vi "CPP-5168-SurfaceCp-Jan2013.vi"() -> (5 "Plug in titles":string[](array[string]), 7 "Plug in values":string[](array[string]))   [LabVIEW 2012]
uses:
  Globals/Meas_global.vi
panel:
  in  "inH20/V":dbl=2.4377 caption="Calibration factor inH20/V"
  in  "Last non-pressure channel":string="HW (HF3)"
  out "Zeroes?":bool
  out "Zeroes":dbl[](array[numeric])
  out "Data":dbl[][](array[numeric]) caption="ZeroedCompensatedCalibratedData" format="%#_3g"
  out "ChannelNames":string[](array[string])
  # "This version doesn't do any window dP calculations"
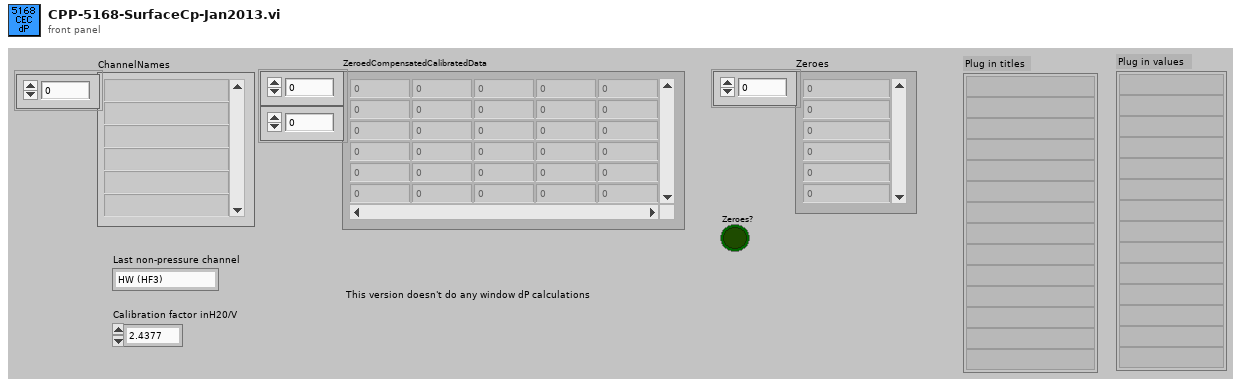
[diagram p1: front panel]
types:
  T1 = typedef "Analysis_info_cluster.ctl" = cluster{"Colour":u32, "Inst type":T2, "Inst name":string, "Symbol":string, "Code name":string, "Extra Info":string, "Inst Array":T3, "Extra Titles":string[], "Extra Values":string[], "U":dbl, "u^2":dbl, "u^3":dbl, "u^4":dbl, "Skew_u":dbl, "Kurt_u":dbl, "Sd Error in Mean":dbl, "% u'/U":dbl, "X":dbl, "Y":dbl, "Z":dbl, "Timescale integral to 25%":dbl, "Sd Error in Variance":dbl, "Calib File":path, "Calib Constants":dbl[], "Output Position":bool, "Full Stats":bool, "Av Sampling Rate":dbl, "Av No of Samples":dbl, "Total Meas Time (s)":dbl, "ADAM Ch Name":string}
  T2 = typedef "Inst_type.ctl" = enum16{"Propeller anemometer", "Raw voltage", "Pressure Transducer", "Pitot-static tube", "Preston tube", "Hot wire", "Cross wire 1", "Cross wire 2", "Generic Linear", "Generic Polynomial", "Generic BackPoly", "Fast FID", "Thermocouple", "Cold wire", "Pulsed Wire", "LDA Vel", "LDA Tran time", "LDA Arr time"}
  T3 = typedef "Instrument_Array.ctl" = enum16{"PWA", "LDA", "Analogue"}
  T4 = typedef "Time_Trace_Cluster.ctl" = cluster{"Weighting":dbl[], "Time (s)":dbl[], "Voltage":dbl[], "Eng Values":dbl[]}
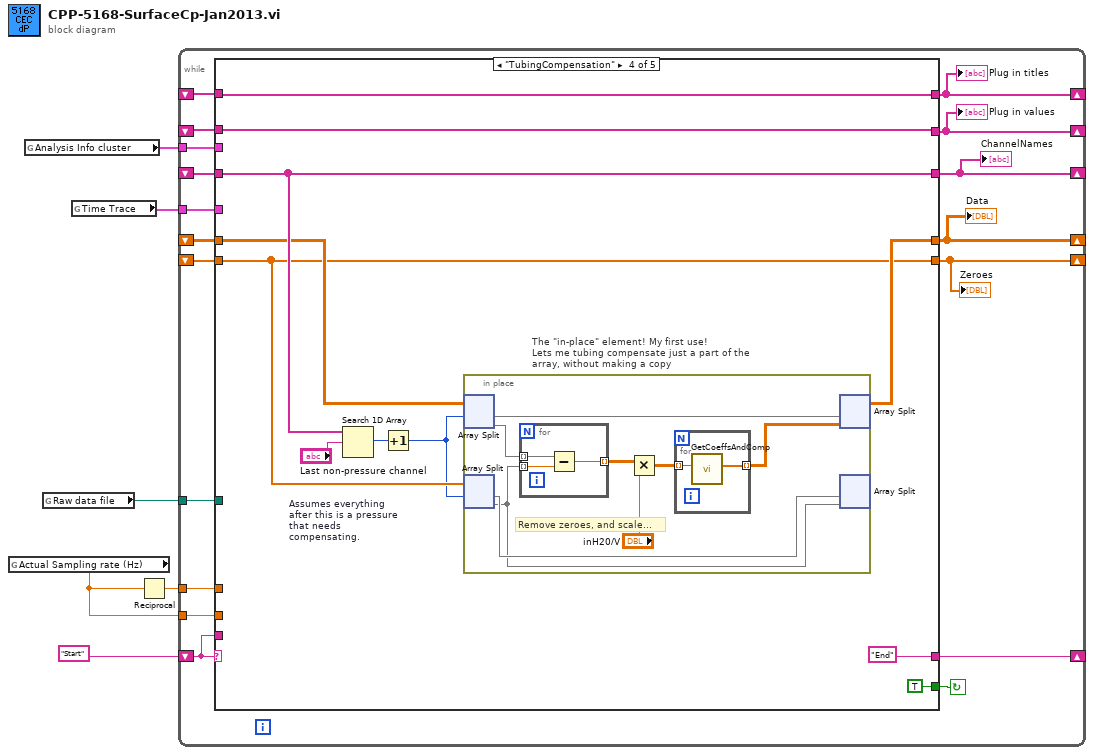
[diagram p0: block diagram]
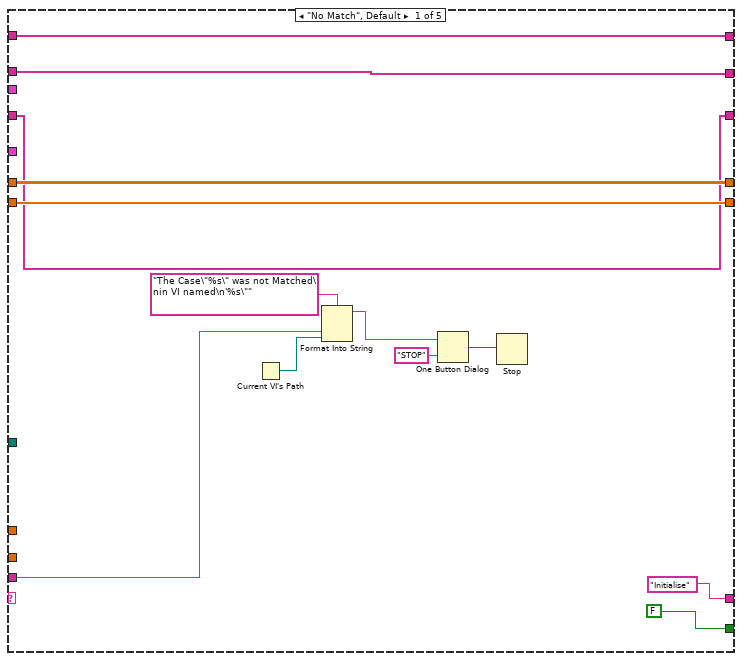
[diagram p2: hidden frame]
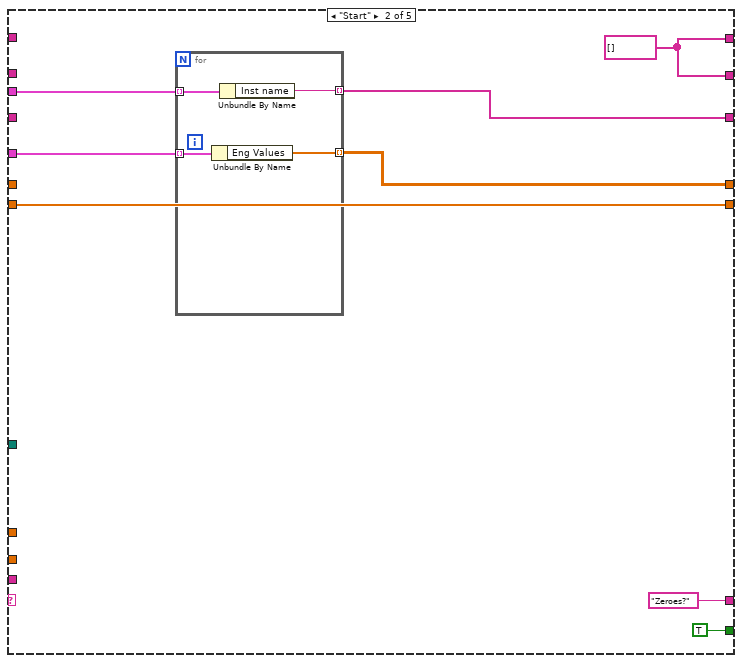
[diagram p3: hidden frame]
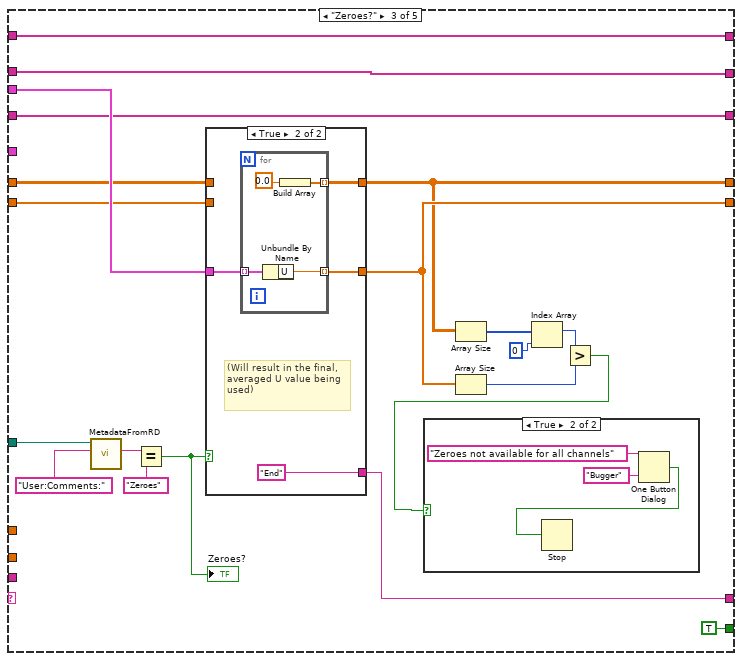
[diagram p4: hidden frame]
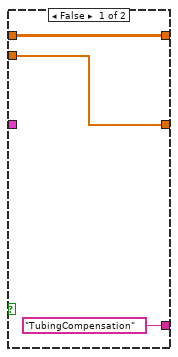
[diagram p6: hidden frame]
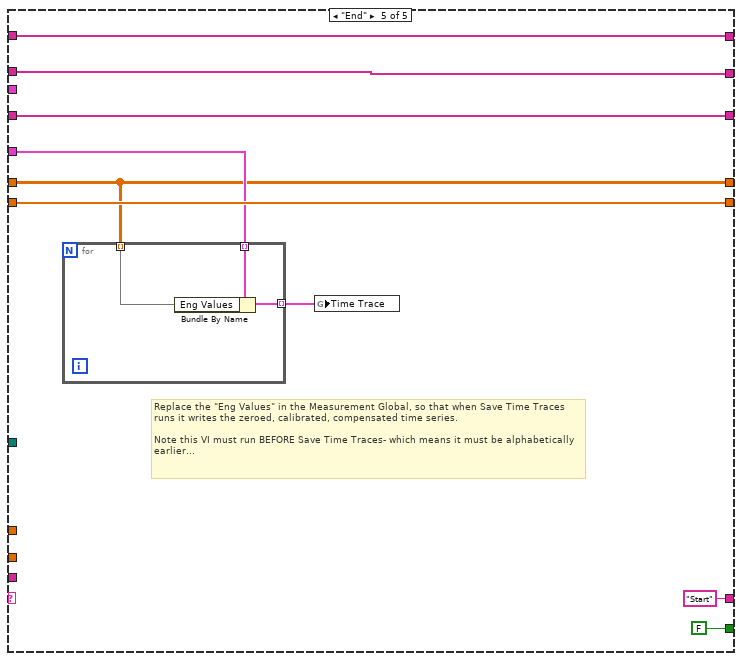
[diagram p7: hidden frame]
diagram:
  n1 = global read "Meas_global.vi" "Actual Sampling rate (Hz)"() -> (w5:dbl)
  n2 = global read "Meas_global.vi" "Analysis Info cluster"() -> (w2:T1[])
  n3 = global read "Meas_global.vi" "Raw data file"() -> (w3:path)
  n4 = global read "Meas_global.vi" "Time Trace"() -> (w1:T4[])
  n5 = Reciprocal(x=w5) -> (1/x=w4:dbl)
  n6 = while {
    shift-left: "Start" -> [w22]
    shift-right: [w23] -> _
    tunnel: w5 -> [w21]
    tunnel: w4 -> [w20]
    tunnel: w3 -> [w17]
    shift-right: [w11] -> _
    shift-left: _ -> [w16]
    shift-right: [w12] -> _
    shift-left: _ -> [w15]
    shift-right: [w14] -> _
    shift-left: _ -> [w13]
    shift-right: [w10] -> _
    shift-left: _ -> [w19]
    tunnel: w2 -> [w9]
    tunnel: w1 -> [w8]
    shift-right: [w7] -> _
    shift-left: _ -> [w18]
    stop <- w24 continue-if-true
    n7 = case shown="\"TubingCompensation\"" w22 {
      tunnel: [FALSE TRUE ("Processing last block?") TRUE ("Processing last block?") TRUE ("Processing last block?") FALSE ("Processing last block?")] -> w24
      tunnel: ["Initialise" "Zeroes?" w61 "End" ("f") "Start" ("f")] -> w23
      tunnel: w22 -> [w32 _ _ _ _]
      tunnel: w21 -> [_ _ _ _ _]
      tunnel: w20 -> [_ _ _ _ _]
      tunnel: w19 -> [w26 _ w50 w86 w109]
      tunnel: w18 -> [w25 _ w52 w90 w108]
      tunnel: w17 -> [_ _ w69 _ _]
      tunnel: w16 -> [w29 _ w67 w88 w114]
      tunnel: [w29 w43 w67 w88 w114] -> w11
      tunnel: [w28 w43 w66 w87 w113] -> w12
      tunnel: w15 -> [w28 _ w66 w87 w113]
      tunnel: [w27 w42 w60 w85 w112] -> w14
      tunnel: w13 -> [w27 w42 w53 w85 w112]
      tunnel: [w26 w40 w51 w89 w109] -> w10
      tunnel: w9 -> [_ w39 w54 _ _]
      tunnel: w8 -> [_ w41 _ _ w111]
      tunnel: [w25 w38 w52 w90 w108] -> w7
      frame "No Match", Default {
        n8 = Current VI's Path() -> (path=w31:path)
        n9 = Format Into String(format string="The Case\"%s\" was not Matched\nin VI named\n'%s\"" ("Format String"), w32, w31) -> (resulting string=w35:string)  [unwired: 2 in, 1 out]
        n10 = One Button Dialog(message=w35, button name ("OK")="STOP") -> (true=w33:bool)
        n11 = Stop(stop? (T)=w33) -> ()
      }
      frame "Start" {
        w43 = string[] []
        n12 = for {
          tunnel: [w48] -> w40 mode=indexing
          tunnel: w41 -> [w49] mode=indexing
          tunnel: w39 -> [w47] mode=indexing
          tunnel: [w46] -> w38 mode=indexing
          n13 = Unbundle By Name(w49) -> ("Eng Values"=w48:dbl[])
          n14 = Unbundle By Name(w47) -> ("Inst name"=w46:string)
        }
      }
      frame "Zeroes?" {
        n15 = call "MetadataFromRD.vi"("ChannelName"="User:Comments:", "Raw data file"=w69) -> ("ValueString"=w64:string)  [unwired: 8 in, 1 out]
        n16 = Equal?(x=w64, y="Zeroes") -> (x = y?=w62:bool)
        "Zeroes?" <- w62
        n17 = case shown="True" w62 {
          tunnel: ["TubingCompensation" ("f") "End" ("f")] -> w61
          tunnel: [w74 w77] -> w60
          tunnel: w54 -> [_ w78]
          tunnel: w53 -> [w74 _]
          tunnel: [w73 w76] -> w51
          tunnel: w50 -> [w73 _]
          frame False {
          }
          frame True {
            # "(Will result in the final, averaged U value being used)"
            n18 = for {
              tunnel: w78 -> [w83] mode=indexing
              tunnel: [w82] -> w77 mode=indexing
              tunnel: [w80] -> w76 mode=indexing
              n19 = Unbundle By Name(w83) -> ("U"=w82:dbl)
              n20 = Build Array(0.0) -> (w80:dbl[])
            }
          }
        }
        n21 = Array Size(array=w51) -> (size(s)=w59:i32[])
        n22 = Array Size(array=w60) -> (size(s)=w58:i32)
        n23 = Index Array(array=w59, index=0) -> (element=w57:i32)
        n24 = Greater?(x=w57, y=w58) -> (0:w55:bool)
        n25 = case shown="True" w55 {
          frame False {
          }
          frame True {
            n26 = One Button Dialog(message="Zeroes not available for all channels", button name ("OK")="Bugger") -> (true=w70:bool)
            n27 = Stop(stop? (T)=w70) -> ()
          }
        }
      }
      frame "TubingCompensation" {
        n28 = Search 1D Array "Assumes everything after this is a pressure that needs compensating."(1D array=w90, element="Last non-pressure channel") -> (index of element=w91:i32)  [unwired: 1 in]
        n29 = Increment(x=w91) -> (x+1=w84:i32)
        n30 = in-place "The \"in-place\" element! My first use!\nLets me tubing compensate just a part of the array, without making a copy" {
          # "Remove zeroes, and scale..."
          n31 = in-place-split #1(w86, w84) -> (w102:dbl[][], w98:dbl[][])
          n32 = in-place-split #2(w85, w84) -> (w96:dbl[], w95:dbl[])
          n33 = for {
            tunnel: [w105] -> w97 mode=indexing
            tunnel: w98 -> [w104] mode=indexing
            tunnel: w95 -> [w103] mode=indexing
            n34 = Subtract(x=w104, y=w103) -> (x-y=w105:dbl[])
          }
          n35 = Multiply(x=w97, y="inH20/V") -> (x*y=w100:dbl[][])
          n36 = for {
            tunnel: w100 -> [w107] mode=indexing
            tunnel: [w106] -> w101 mode=indexing
            n37 = call "GetCoeffsAndComp.vi"("mutedData"=w107) -> ("boostedData"=w106:dbl[])  [unwired: 10 in]
          }
          n38 = in-place-split #1(w102, w101) -> (w89:dbl[][])  [unwired: 1 out]
          n39 = in-place-split #2(w96, w95) -> ()  [unwired: 2 out]
        }
      }
      frame "End" {
        # "Replace the \"Eng Values\" in the Measurement Global, so that when Save Time Traces runs it writes the zeroed, calibrated, compensated time series.\n\nNote this VI must run BEFORE Save Time Traces- which means it must be alphabetically earlier..."
        n40 = for {
          tunnel: w111 -> [w119] mode=indexing
          tunnel: [w118] -> w110 mode=indexing
          tunnel: w109 -> [w117] mode=indexing
          n41 = Bundle By Name(cluster=w119, "Eng Values"=w117) -> (w118:T4)
        }
        n42 = global write "Meas_global.vi" "Time Trace"(w110) -> ()
      }
    }
    "Plug in values" <- w12
    "Plug in titles" <- w11
    "Data" <- w10
    "Zeroes" <- w14
    "ChannelNames" <- w7
  }
